vi "Compile Arduino.vi"(8 "Error In":errorcluster, 11 "input filename":path) -> (0 "Error Out":errorcluster, 2 "standard error":string, 3 "standard output":string)   [LabVIEW 2014]
panel:
  out "concatenated string":string
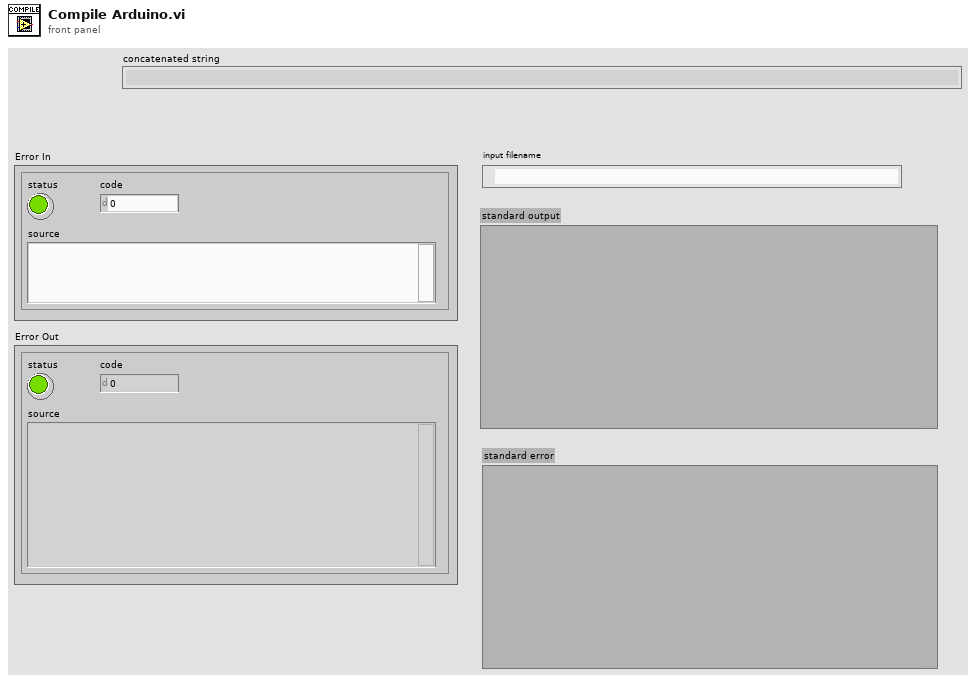
[diagram p1: front panel]
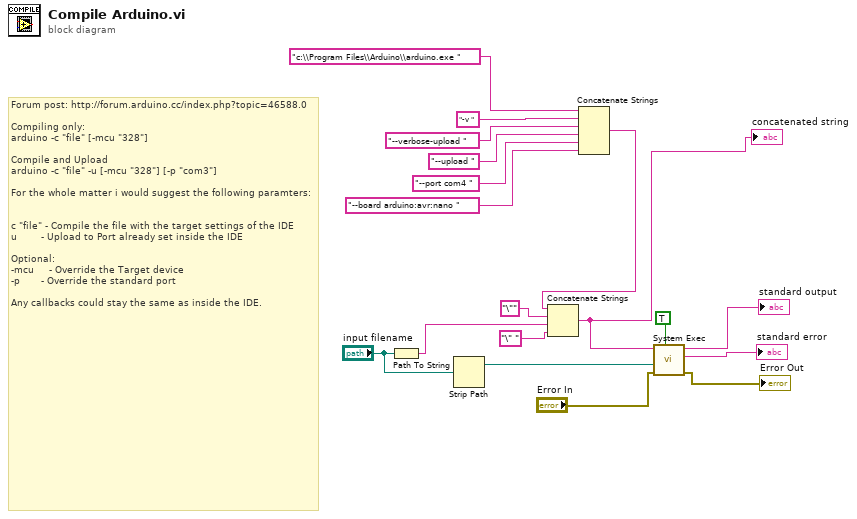
[diagram p0: block diagram]
diagram:
  # "Forum post: http://forum.arduino.cc/index.php?topic=46588.0 \n\nCompiling only:\narduino -c \"file\" [-mcu \"328\"]\n\nCompile and Upload\narduino -c \"file\" -u [-mcu \"328\"] [-p \"com3\"]\n\nFor the whole matter i would suggest the following paramters:\n\n\nc \"file\" - Compile the file with the target settings of the IDE\nu        - Upload to Port already set inside the IDE\n\nOptional:\n-mcu     - Override the Target device\n-p       - Override the standard port\n\nAny callbacks could stay the same as inside the IDE."
  n1 = Path To String(path="input filename") -> (string=w12:string)
  n2 = Strip Path(path="input filename") -> (stripped path=w3:path)  [unwired: 1 out]
  n3 = Concatenate Strings("c:\\Program Files\\Arduino\\arduino.exe " ("command line"), "-v " ("string"), "--verbose-upload " ("string"), "--upload " ("string"), "--port com4 " ("string"), "--board arduino:avr:nano " ("string")) -> (w10:string)
  n4 = Concatenate Strings(w10, "\"" ("string"), w12, "\" " ("string")) -> (w1:string)
  "concatenated string" <- w1
  n5 = call <vilib>:"System Exec.vi"("wait until completion? (T)"=TRUE, "error in (no error)"="Error In", "working directory"=w3, "command line"=w1) -> ("error out"=→"Error Out":errorcluster, "standard error"=→"standard error":string, "standard output"=→"standard output":string)  [unwired: 4 in, 1 out]
